vi "DMA Settings.vi"(6 "Action":T3, 8 "error in (no error)":errorcluster, 10 "DMA Settings":T1={"Number of Channels"=0, "Delacing Scheme"=enum."Interlaced", "Update Rate"=1, "dt"=0.0001} {"dt" format="%#_p"; "Update Rate" items=["1 Hz"=1, "2 Hz"=2, "5 Hz"=5, "10 Hz"=10]}, 11 "Item Ref":T4 format="%.0x") -> (0 "error out":errorcluster, 2 "DMA Settings":T1={"Number of Channels"=1, "Delacing Scheme"=enum."Interlaced", "Update Rate"=1000, "dt"=1000.0} {"dt" format="%#_p"; "Update Rate" items=["1 Hz"=1, "2 Hz"=2, "5 Hz"=5, "10 Hz"=10]}, 3 "Item Ref out":T4=18446744073709551615 format="%.0x")   [LabVIEW 2015, in "FPGA Addon Shared.lvlib"]
uses:
  FPGA Addon Shared.lvlib
  DMA Settings.ctl
  Delacing Scheme.ctl
  <vilib>/NI Veristand/Custom Device API/Custom Device Item Ref.ctl
  FG Action.ctl
  <vilib>/NI Veristand/Custom Device API/Set Item Property (Double).vi
  <vilib>/NI Veristand/Custom Device API/Set Item Property (U32).vi
  <vilib>/NI Veristand/Custom Device API/Get Item Property (Double).vi
  <vilib>/NI Veristand/Custom Device API/Get Item Property (U32).vi
  Constants.vi
  <vilib>/NI VeriStand/Custom Device API/Custom Device API.lvlib
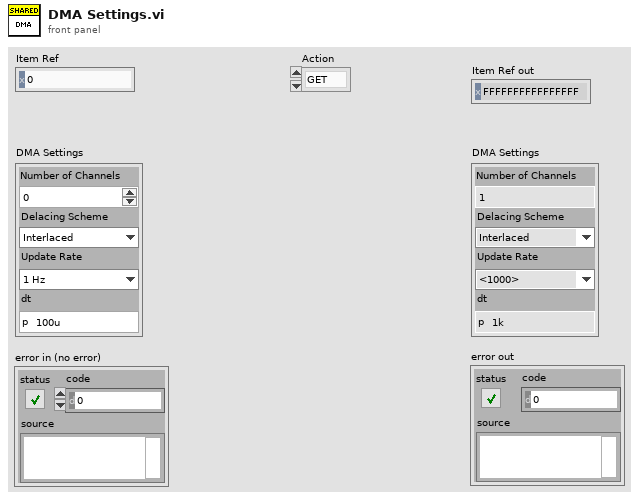
[diagram p1: front panel]
types:
  T1 = typedef "FPGA Addon Shared.lvlib/DMA Settings.ctl" = cluster{"Number of Channels":u8, "Delacing Scheme":T2, "Update Rate":u32, "dt":dbl}
  T2 = typedef "FPGA Addon Shared.lvlib/Delacing Scheme.ctl" = enum8{"Interlaced"}
  T3 = typedef "FPGA Addon Shared.lvlib/FG Action.ctl" = enum8{"GET", "SET"}
  T4 = typedef "Custom Device API.lvlib/Custom Device Item Ref.ctl" = u64
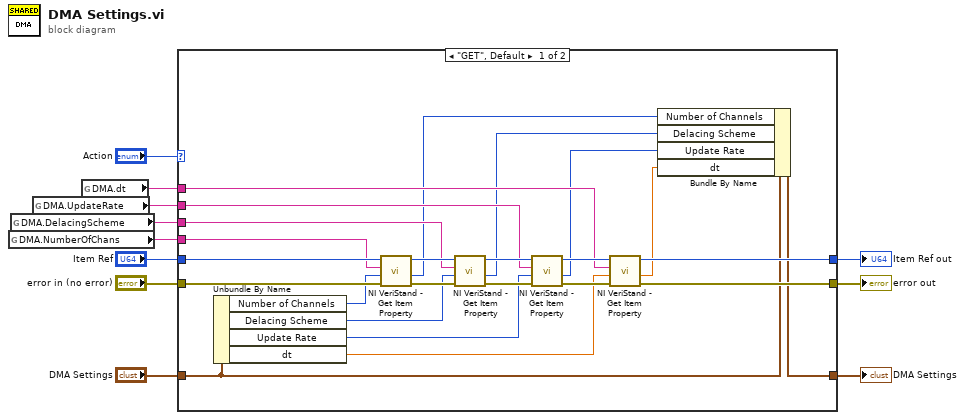
[diagram p0: block diagram]
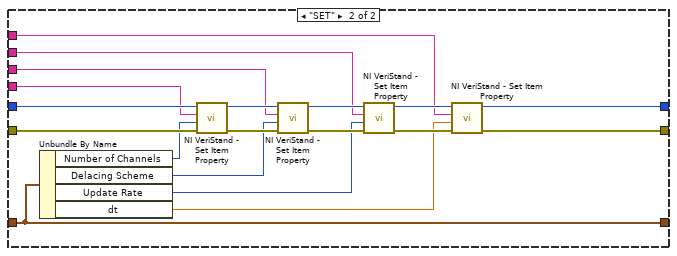
[diagram p2: hidden frame]
diagram:
  n1 = global read "Constants.vi" "DMA.NumberOfChans"() -> (w5:string)
  n2 = global read "Constants.vi" "DMA.DelacingScheme"() -> (w3:string)
  n3 = global read "Constants.vi" "DMA.UpdateRate"() -> (w2:string)
  n4 = global read "Constants.vi" "DMA.dt"() -> (w1:string)
  n5 = case shown="\"GET\", Default" "Action" {
    tunnel: "error in (no error)" -> [w35 w54]
    tunnel: "Item Ref" -> [w34 w53]
    tunnel: "DMA Settings" -> [w13 w36]
    tunnel: [w29 w45] -> w11
    tunnel: [w28 w46] -> w7
    tunnel: [w12 w36] -> w4
    tunnel: w5 -> [w33 w52]
    tunnel: w3 -> [w24 w42]
    tunnel: w2 -> [w23 w41]
    tunnel: w1 -> [w22 w40]
    frame "GET", Default {
      n6 = Unbundle By Name(w13) -> ("Number of Channels"=w18:u8, "Delacing Scheme"=w19:T2, "Update Rate"=w20:u32, "dt"=w21:dbl)
      n7 = call-poly <vilib>:"NI VeriStand - Get Item Property.vi"("error in (no error)"=w35, "Default Value"=w18, "Property Name"=w33, "Item Ref in"=w34) -> ("error out"=w32:errorcluster, "Value"=w17:u32, "Item Ref out"=w25:T4)  [unwired: 4 in, 1 out]
      n8 = call-poly <vilib>:"NI VeriStand - Get Item Property.vi"("error in (no error)"=w32, "Default Value"=w19, "Property Name"=w24, "Item Ref in"=w25) -> ("error out"=w31:errorcluster, "Value"=w16:u32, "Item Ref out"=w26:T4)  [unwired: 4 in, 1 out]
      n9 = call-poly <vilib>:"NI VeriStand - Get Item Property.vi"("error in (no error)"=w31, "Default Value"=w20, "Property Name"=w23, "Item Ref in"=w26) -> ("error out"=w30:errorcluster, "Value"=w15:u32, "Item Ref out"=w27:T4)  [unwired: 4 in, 1 out]
      n10 = call-poly <vilib>:"NI VeriStand - Get Item Property.vi"("error in (no error)"=w30, "Default Value"=w21, "Property Name"=w22, "Item Ref in"=w27) -> ("error out"=w29:errorcluster, "Value"=w14:dbl, "Item Ref out"=w28:T4)  [unwired: 4 in, 1 out]
      n11 = Bundle By Name(cluster=w13, "Number of Channels"=w17, "Delacing Scheme"=w16, "Update Rate"=w15, "dt"=w14) -> (w12:T1)
    }
    frame "SET" {
      n12 = Unbundle By Name(w36) -> ("Number of Channels"=w51:u8, "Delacing Scheme"=w39:T2, "Update Rate"=w38:u32, "dt"=w37:dbl)
      n13 = call-poly <vilib>:"NI VeriStand - Set Item Property.vi"("error in (no error)"=w54, "Value"=w51, "Property Name"=w52, "Item Ref in"=w53) -> ("error out"=w49:errorcluster, "Item Ref out"=w50:T4)  [unwired: 5 in, 1 out]
      n14 = call-poly <vilib>:"NI VeriStand - Set Item Property.vi"("error in (no error)"=w49, "Value"=w39, "Property Name"=w42, "Item Ref in"=w50) -> ("error out"=w43:errorcluster, "Item Ref out"=w48:T4)  [unwired: 5 in, 1 out]
      n15 = call-poly <vilib>:"NI VeriStand - Set Item Property.vi"("error in (no error)"=w43, "Value"=w38, "Property Name"=w41, "Item Ref in"=w48) -> ("error out"=w44:errorcluster, "Item Ref out"=w47:T4)  [unwired: 5 in, 1 out]
      n16 = call-poly <vilib>:"NI VeriStand - Set Item Property.vi"("error in (no error)"=w44, "Value"=w37, "Property Name"=w40, "Item Ref in"=w47) -> ("error out"=w45:errorcluster, "Item Ref out"=w46:T4)  [unwired: 5 in, 1 out]
    }
  }
  "error out" <- w11
  "Item Ref out" <- w7
  "DMA Settings" <- w4
